vi "Dequeue4Elements.vi"() -> (3 "Data Out":i32[](array[numeric]))   [LabVIEW 2020]
uses:
  <vilib>/rvi/DataTransferAndStorage/Container/Common/niFpgaContainerExecOnDevCompGetState.vi
  <vilib>/rvi/Emulation/niFpgaEmulationIsFPGAContextNoSignature.vi
  <vilib>/rvi/Emulation/niFpgaSctlEmulationGetInTimedLoop.vi
  <vilib>/rvi/errors/niFpgaSetErrorForExecOnDevCompSimple.vi
  <vilib>/rvi/eio/common/nirviEmuReportErrorAndStop.vi
  <vilib>/rvi/DataTransferAndStorage/Container/Common/niFpgaContainerGetUniqueNameForEmu.vi
  <vilib>/rvi/FIFO/Fifo_Resource/nirvififoEmulationSetSize.vi
  <vilib>/rvi/FIFO/Fifo_Resource/nirviFifoEmulationQueueMgr.vi
  <instcachedir>/0/nirviFifoEmulationQueueMgr_E5CAEC123FF24DC58D834DCA3CDAA9B5.lvgen/nirviFifoEmulationQueueMgr_E5CAEC123FF24DC58D834DCA3CDAA9B5_009.vi
  <vilib>/rvi/FIFO/Fifo_Resource/nirvififoEmulationDetermineInputValidOut.vi
  <vilib>/rvi/FIFO/Fifo_Resource/nirvififoEmulationCreateLock.vi
  <vilib>/rvi/Emulation/niFpgaProcessEmulError.vi
  <vilib>/rvi/FIFO/Fifo_Resource/nirvififoEmulationObtainLock.vi
  <vilib>/rvi/FIFO/Fifo_Resource/nirvififoEmulationReleaseLock.vi
  <vilib>/rvi/occurrence/nirviWaitOnOccurrenceBase.vi
  <vilib>/rvi/errors/nirviReportUnexpectedCaseInternalError.vi
  <vilib>/rvi/errors/nirviReportUnexpectedCaseInternalError (U32).vi
  <vilib>/Utility/error.llb/Clear Errors.vi
  <vilib>/rvi/interface/RandomDataEmulation/niFpgaRandomDataHandleErrors.vi
  <vilib>/rvi/DataTransferAndStorage/Container/XNode/niFpgaContainer.xnode
  <vilib>/rvi/FIFO/Fifo_Resource/niFpgaFifoEmulationRefIn.vi
  <vilib>/rvi/FIFO/Fifo_Resource/nirvififoEmulationRead.vi
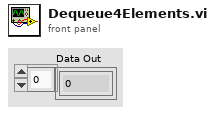
[diagram p1: front panel]
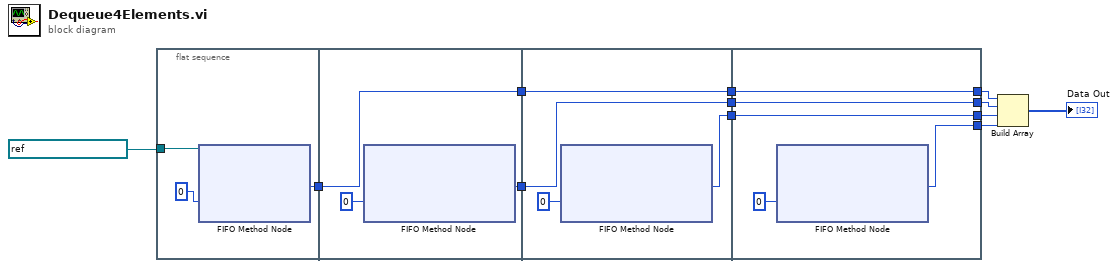
[diagram p0: block diagram]
diagram:
  n1 = flat-sequence {
    tunnel: refnum<k21> "AveragingFIFO-A" ("FIFO In") -> [w14]
    tunnel: [w13] -> w7
    tunnel: [w17] -> w10
    tunnel: [w16] -> w8
    tunnel: w7 -> [w16]
    tunnel: [w21] -> w12
    tunnel: [w20] -> w11
    tunnel: w10 -> [w20]
    tunnel: [w19] -> w9
    tunnel: w8 -> [w19]
    tunnel: [w26] -> w3
    tunnel: [w25] -> w4
    tunnel: w12 -> [w25]
    tunnel: w11 -> [w24]
    tunnel: [w24] -> w5
    tunnel: [w23] -> w6
    tunnel: w9 -> [w23]
    frame #0 {
      n2 = xnode ("FIFO Method Node")("Timeout"=0, "FIFO In"=w14) -> ("Element"=w13:i32)  [unwired: 2 out]
    }
    frame #1 {
      n3 = xnode ("FIFO Method Node")("Timeout"=0) -> ("Element"=w17:i32)  [unwired: 1 in, 2 out]
    }
    frame #2 {
      n4 = xnode ("FIFO Method Node")("Timeout"=0) -> ("Element"=w21:i32)  [unwired: 1 in, 2 out]
    }
    frame #3 {
      n5 = xnode ("FIFO Method Node")("Timeout"=0) -> ("Element"=w26:i32)  [unwired: 1 in, 2 out]
    }
  }
  n6 = Build Array(w6, w5, w4, w3) -> (→"Data Out":i32[])
